vi "index Values of G.vi"() -> ()   [LabVIEW 2022 SP3]
panel:
  in  "index values of G":i32[](array[numeric])
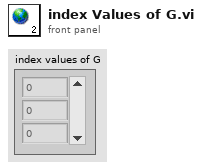
[diagram p1: front panel]
diagram:
